vi "DataLog Example Server.vi"   [LabVIEW 2012]
doc: "This is the top-level VI that starts a server application. It bootstraps LuaVIEW and hands over control to a series of initialisation scripts that define what the application does. The first script is named \"bootstrap.lua\" and is read from a \"resources\" directory located respectively in the same directory as this VI or inside the application directory, depending on whether this VI is run under the development system or as a built application.\n\nWhen building a server application, this is the main VI to include in the build. In addition you will need to include any dynamically loaded VIs, functions, modules, and plug-ins that are used by the server's scripts."
uses:
  clientsrv/subvis/private/glb_ClientSrv Globals.vi
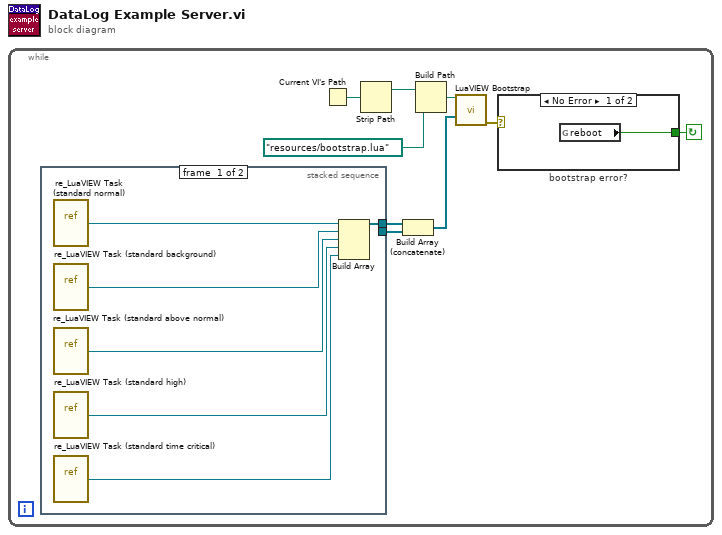
[diagram p0: block diagram]
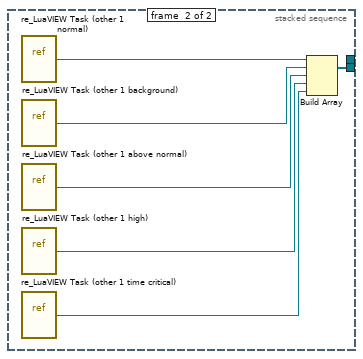
[diagram p2: hidden frame]
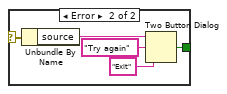
[diagram p3: hidden frame]
diagram:
  n1 = while {
    stop <- w5 continue-if-true
    n2 = stacked-sequence {
      tunnel: [w10 _] -> w4
      tunnel: [_ w16] -> w3
      frame #0 {
        n3 = vi-ref "re_LuaVIEW Task (standard normal).vi"() -> ("vi reference"=w15:refnum<vi>)
        n4 = vi-ref "re_LuaVIEW Task (standard background).vi"() -> ("vi reference"=w14:refnum<vi>)
        n5 = vi-ref "re_LuaVIEW Task (standard above normal).vi"() -> ("vi reference"=w13:refnum<vi>)
        n6 = vi-ref "re_LuaVIEW Task (standard high).vi"() -> ("vi reference"=w12:refnum<vi>)
        n7 = vi-ref "re_LuaVIEW Task (standard time critical).vi"() -> ("vi reference"=w11:refnum<vi>)
        n8 = Build Array(w15, w14, w13, w12, w11) -> (w10:refnum<vi>[])
      }
      frame #1 {
        n9 = vi-ref "re_LuaVIEW Task (other 1 normal).vi"() -> ("vi reference"=w21:refnum<vi>)
        n10 = vi-ref "re_LuaVIEW Task (other 1 background).vi"() -> ("vi reference"=w20:refnum<vi>)
        n11 = vi-ref "re_LuaVIEW Task (other 1 above normal).vi"() -> ("vi reference"=w19:refnum<vi>)
        n12 = vi-ref "re_LuaVIEW Task (other 1 high).vi"() -> ("vi reference"=w18:refnum<vi>)
        n13 = vi-ref "re_LuaVIEW Task (other 1 time critical).vi"() -> ("vi reference"=w17:refnum<vi>)
        n14 = Build Array(w21, w20, w19, w18, w17) -> (w16:refnum<vi>[])
      }
    }
    n15 = Current VI's Path() -> (path=w1:path)
    n16 = Strip Path(path=w1) -> (stripped path=w7:path)  [unwired: 1 out]
    n17 = Build Array (concatenate)(w4, w3) -> (w2:refnum<vi>[])
    n18 = Build Path(base path=w7, name or relative path=path "resources/bootstrap.lua" ("script file or name (no name)")) -> (appended path=w8:path)
    n19 = call "LuaVIEW Bootstrap.vi"("script file or name (no name)"=w8, "task alternatives (default)"=w2) -> ("error out"=w6:errorcluster)  [unwired: 13 in]
    n20 = case "bootstrap error?" shown="No Error" w6 {
      selector: w6 -> [_ w27]
      tunnel: [w22 w23] -> w5
      frame No Error {
        n21 = global read "glb_ClientSrv Globals.vi" "reboot"() -> (w22:bool)
      }
      frame Error {
        n22 = Unbundle By Name(w27) -> ("source"=w26:string)
        n23 = Two Button Dialog(message=w26, 1:"Exit" ("F button name (\"Cancel\")"), 2:"Try again" ("T button name (\"OK\")")) -> (T button?=w23:bool)
      }
    }
  }
